vi "write pockels cell task.vi"(8 "error in (no error)":errorcluster, 11 "Waveform in":refnum<class "Waveform.lvclass">) -> (0 "error out":errorcluster, 3 "Waveform out":refnum<class "Waveform.lvclass">)   [LabVIEW 2012, in "Waveform.lvclass"]
uses:
  Waveform.lvclass
  PC_wavelength.ctl
  Waveform.lvclass/Waveform.ctl
  <vilib>/DAQmx/write.llb/DAQmx Write (Analog DBL 1Chan 1Samp).vi
  <vilib>/DAQmx/miscellaneous.llb/DAQmx Fill In Error Info.vi
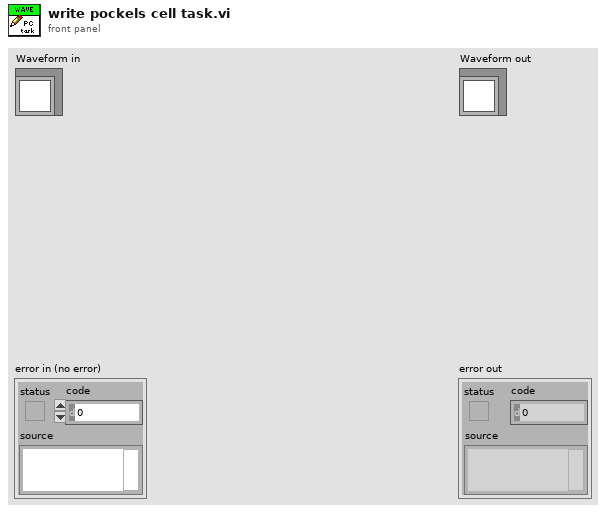
[diagram p1: front panel]
types:
  T1 = typedef "PC_wavelength.ctl" = dbl
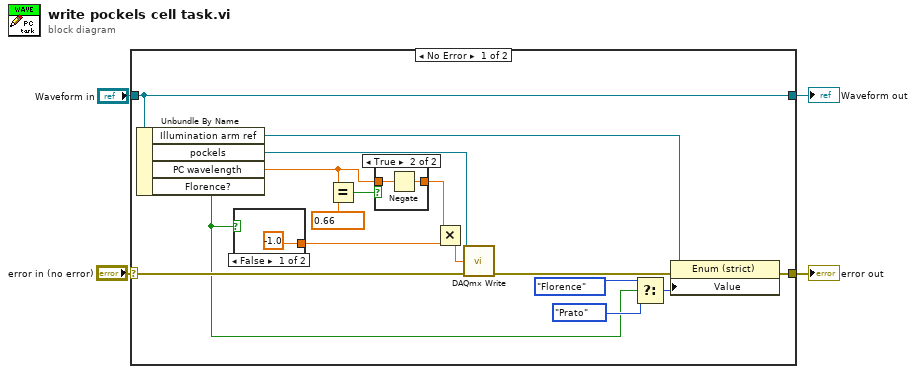
[diagram p0: block diagram]
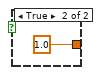
[diagram p3: hidden frame]
diagram:
  n1 = case shown="No Error" "error in (no error)" {
    selector: "error in (no error)" -> [w19 w27]
    tunnel: [w9 w27] -> w3
    tunnel: [w20 w26] -> w1
    tunnel: "Waveform in" -> [w20 w26]
    frame No Error {
      w15 = T1 0.66 items=["405nm"=0.48, "445nm"=0.52, "491nm"=0.58, "515nm"=0.6, "561nm"=0.66] ("y")
      n2 = Unbundle By Name(w20) -> ("Illumination arm ref"=w11:refnum<vi>, "pockels"=w18:refnum<k21>, "PC wavelength"=w13:T1, "Florence?"=w5:bool)
      n3 = case shown="False" w5 {
        tunnel: [-1.0 1.0] -> w17
        frame False {
        }
        frame True {
        }
      }
      n4 = Equal?(x=w13, y=w15) -> (x = y?=w14:bool)
      n5 = case shown="True" w14 {
        tunnel: w13 -> [w21 w23]
        tunnel: [w21 w22] -> w12
        frame False {
        }
        frame True {
          n6 = Negate(x=w23) -> (-x=w22:T1)
        }
      }
      n7 = Multiply(x=w12, y=w17) -> (x*y=w16:T1)
      n8 = call-poly <vilib>:"DAQmx Write.vi"("task/channels in"=w18, "data"=w16, "error in"=w19) -> ("error out"=w10:errorcluster)  [unwired: 10 in, 2 out]
      n9 = Select(t=enum16{"Florence", "Prato"}."Florence" ("Value"), s=w5, f=enum16{"Florence", "Prato"}."Prato" ("Value")) -> (s? t:f=w8:enum16{"Florence", "Prato"})
      n10 = property class="Enum (strict)"(reference=w11, error in=w10, "Value"=w8) -> (error out=w9:errorcluster)  [unwired: 1 out]
    }
    frame Error {
    }
  }
  "error out" <- w3
  "Waveform out" <- w1
